vi "Save_Stats_for_Each_Block.vi"() -> (5 "Plug in titles":string[](array[string]), 7 "Plug in values":string[](array[string]))   [LabVIEW 2010]
uses:
  Globals/Meas_global.vi
  Globals/Plug_in_data_global.vi
  Globals/LDA_meas_global_1.vi
  <vilib>/Analysis/NI_AALBase.lvlib
panel:
  in  "Output Directory":path
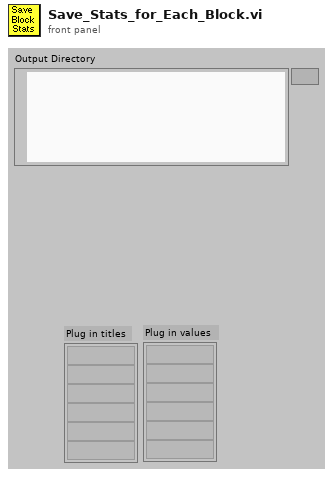
[diagram p1: front panel]
types:
  T1 = typedef "Analysis_info_cluster.ctl" = cluster{"Colour":u32, "Inst type":T2, "Inst name":string, "Symbol":string, "Code name":string, "Extra Info":string, "Inst Array":T3, "Index":i32, "Voltage Index":i32, "Extra Titles":string[], "Extra Values":string[]}
  T2 = typedef "Inst_type.ctl" = enum16{"Propeller anemometer", "Raw voltage", "Pressure Transducer", "Pitot-static tube", "Preston tube", "Hot wire", "Cross wire 1", "Cross wire 2", "Generic Linear", "Generic Polynomial", "Generic BackPoly", "Fast FID", "Thermocouple", "Cold wire", "Pulsed Wire", "LDA Vel", "LDA Tran time", "LDA Arr time"}
  T3 = typedef "Instrument_Array.ctl" = enum16{"PWA", "LDA", "Analogue"}
  T4 = enum32{"existing file", "new file", "new or existing file", "existing dir", "new dir", "new or existing dir", "existing file (use LLBs)", "new file (use LLBs)", "new or existing file (use LLBs)", "new or existing file or directory (use LLBs)"}
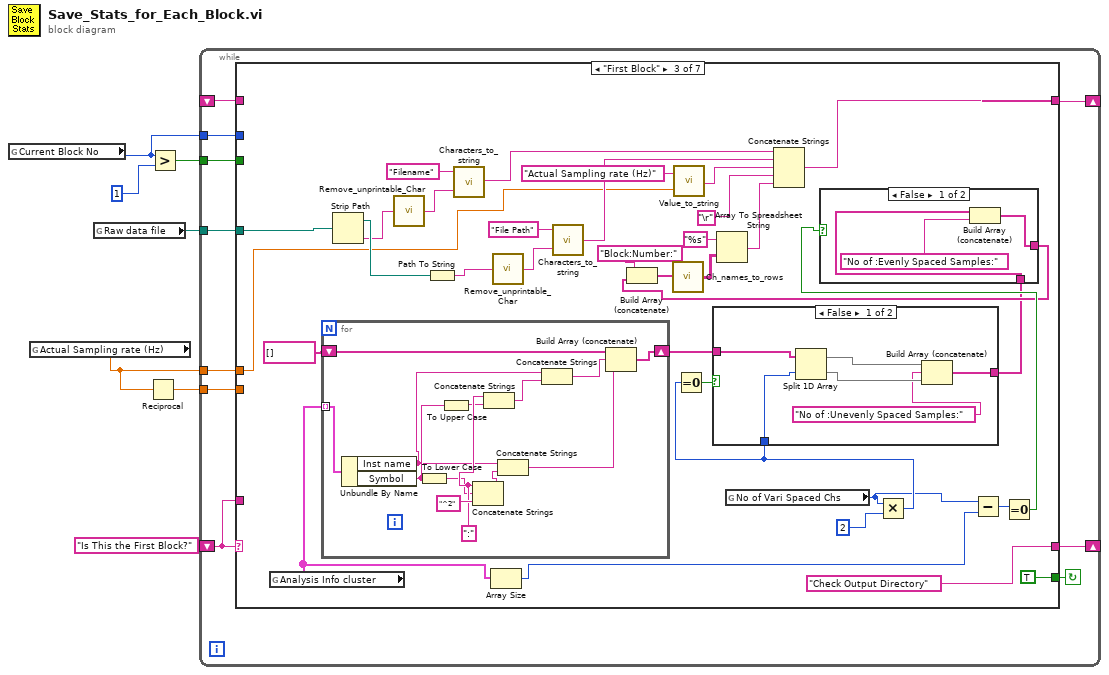
[diagram p0: block diagram]
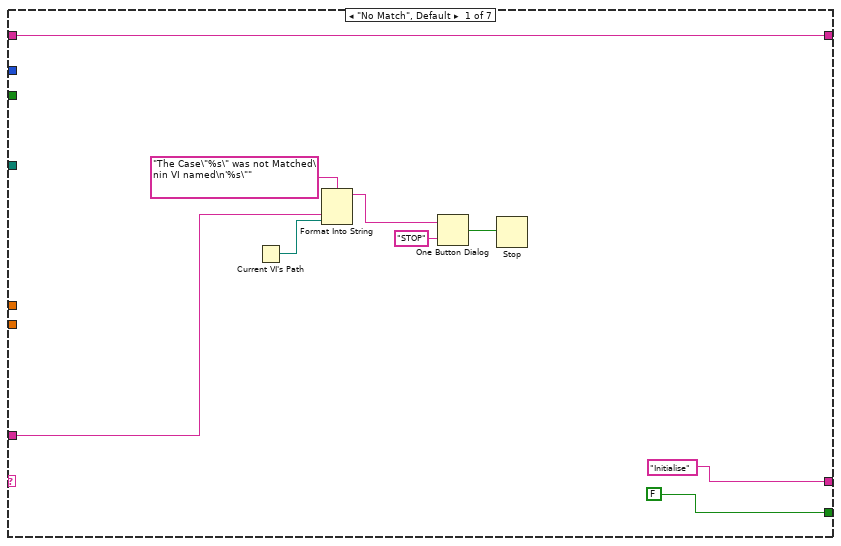
[diagram p2: hidden frame]
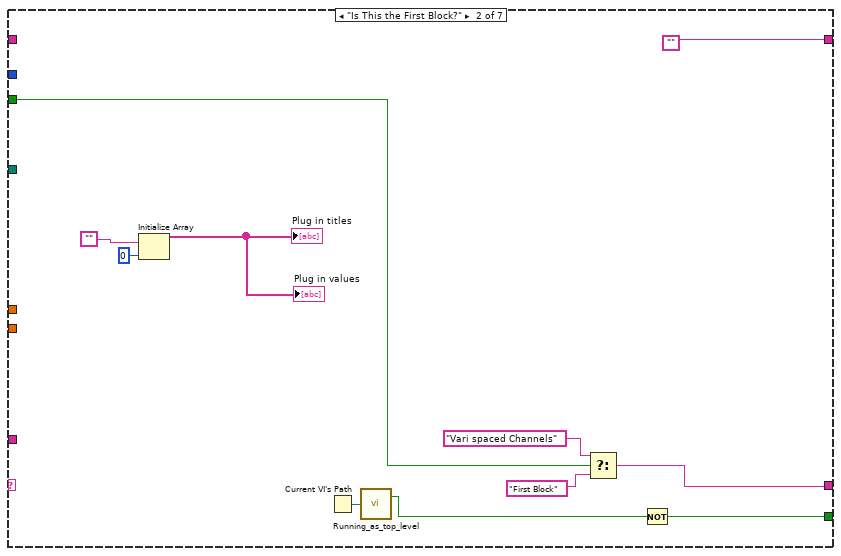
[diagram p3: hidden frame]
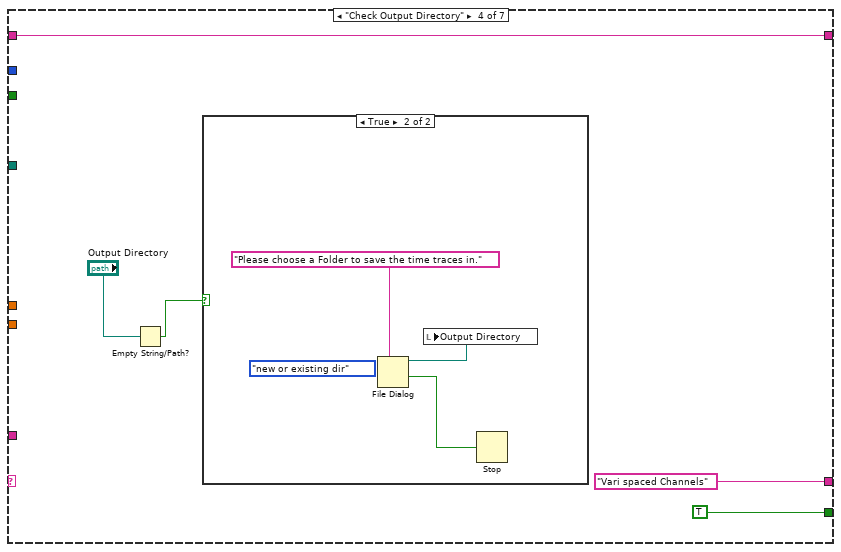
[diagram p6: hidden frame]
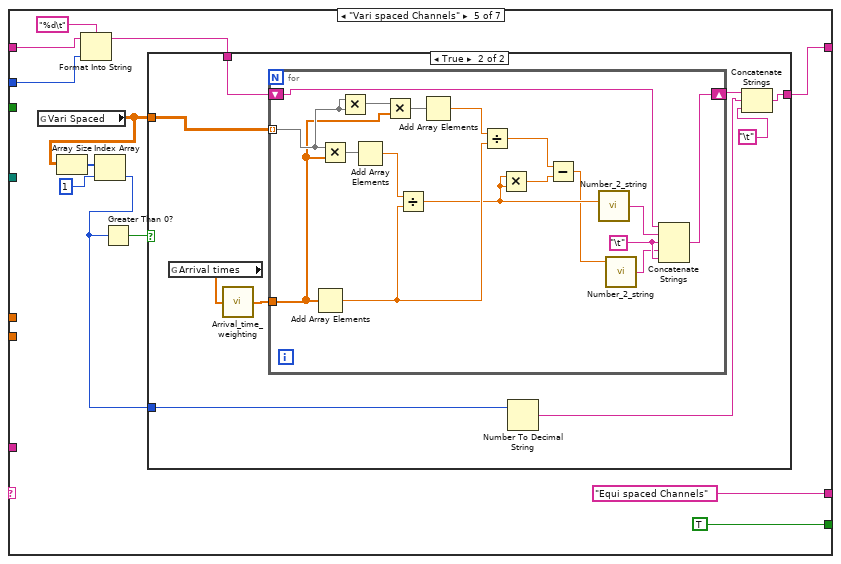
[diagram p8: hidden frame]
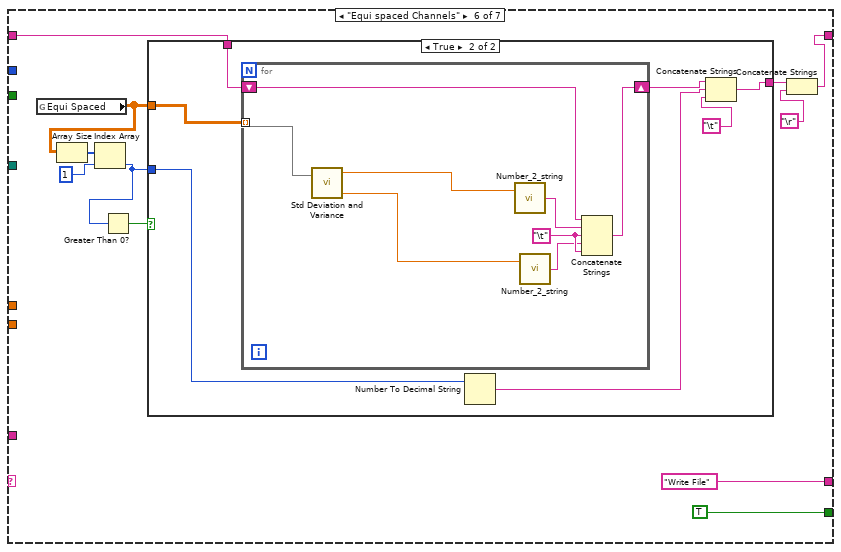
[diagram p10: hidden frame]
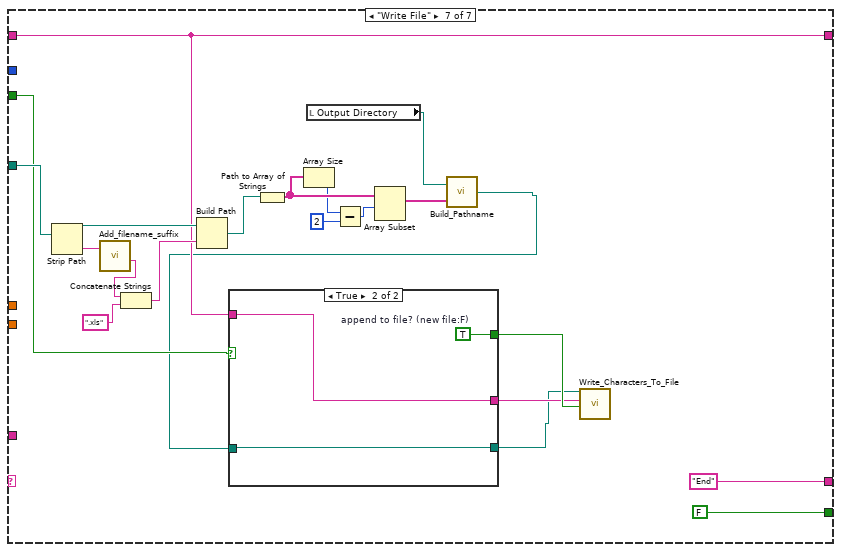
[diagram p12: hidden frame]
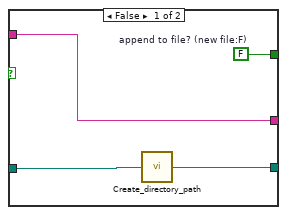
[diagram p13: hidden frame]
diagram:
  n1 = global read "Meas_global.vi" "Current Block No"() -> (w1:i32)
  n2 = global read "Meas_global.vi" "Actual Sampling rate (Hz)"() -> (w2:dbl)
  n3 = global read "Meas_global.vi" "Raw data file"() -> (w6:path)
  n4 = Reciprocal(x=w2) -> (1/x=w5:dbl)
  n5 = Greater?(x=w1, y=1) -> (0:w3:bool)
  n6 = while {
    shift-left: "Is This the First Block?" -> [w15]
    shift-right: [w16] -> _
    shift-right: [w13] -> _
    shift-left: _ -> [w12]
    tunnel: w6 -> [w14]
    tunnel: w5 -> [w11]
    tunnel: w3 -> [w10]
    tunnel: w2 -> [w9]
    tunnel: w1 -> [w8]
    stop <- w17 continue-if-true
    n7 = case shown="\"First Block\"" w15 {
      tunnel: [FALSE w27 TRUE TRUE TRUE TRUE FALSE] -> w17
      tunnel: ["Initialise" w36 "Check Output Directory" ("t") "Vari spaced Channels" ("t") "Equi spaced Channels" "Write File" "End" ("t")] -> w16
      tunnel: w15 -> [w21 _ _ _ _ _ _]
      tunnel: w14 -> [_ _ w60 _ _ _ w186]
      tunnel: [w18 "" w59 w98 w113 w145 w181] -> w13
      tunnel: w12 -> [w18 _ _ w98 w108 w151 w181]
      tunnel: w11 -> [_ _ _ _ _ _ _]
      tunnel: w10 -> [_ w34 _ _ _ _ w182]
      tunnel: w9 -> [_ _ w53 _ _ _ _]
      tunnel: w8 -> [_ _ _ _ w107 _ _]
      frame "No Match", Default {
        n8 = Current VI's Path() -> (path=w20:path)
        n9 = Format Into String(format string="The Case\"%s\" was not Matched\nin VI named\n'%s\"" ("Format String"), w21, w20) -> (resulting string=w24:string)  [unwired: 2 in, 1 out]
        n10 = One Button Dialog(message=w24, button name ("OK")="STOP") -> (true=w22:bool)
        n11 = Stop(stop? (T)=w22) -> ()
      }
      frame "Is This the First Block?" {
        n12 = Initialize Array("", 0) -> (→"Plug in values" →"Plug in titles":string[])
        n13 = Current VI's Path() -> (path=w29:path)
        n14 = call "Running_as_top_level.vi"("Vi path name"=w29) -> ("Top Level"=w28:bool)  [unwired: 1 out]
        n15 = Select(t="Vari spaced Channels", s=w34, f="First Block") -> (s? t:f=w36:string)
        n16 = Not(x=w28) -> (.not. x?=w27:bool)
      }
      frame "First Block" {
        n17 = global read "Meas_global.vi" "Analysis Info cluster"() -> (w45:T1[])
        n18 = for {
          tunnel: w45 -> [w95] mode=indexing
          shift-right: [w83] -> w50
          shift-left: string[] [] -> [w86]
          w91 = ":" ("string")
          n19 = Unbundle By Name(w95) -> ("Inst name"=w87:string, "Symbol"=w89:string)
          n20 = To Lower Case(string=w89) -> (all lower case string=w90:string)
          n21 = To Upper Case(1:w89) -> (0:w88:string)
          n22 = Concatenate Strings(w91, w90, "^2") -> (w93:string)
          n23 = Concatenate Strings(w91, w88) -> (w92:string)
          n24 = Concatenate Strings(w87, w93) -> (w84:string)
          n25 = Concatenate Strings(w87, w92) -> (w85:string)
          n26 = Build Array (concatenate)(w86, w85, w84) -> (w83:string[])
        }
        n27 = Strip Path(path=w60) -> (stripped path=w67:path, name=w63:string)
        n28 = call "Remove_unprintable_Char.vi"("Input String"=w63) -> ("Output String"=w64:string)
        n29 = Path To String(path=w67) -> (string=w68:string)
        n30 = call "Characters_to_string.vi"("Characters to write"=w64, "Label for characters"="Filename") -> ("Output string"=w69:string)
        n31 = Array Size(array=w45) -> (size(s)=w44:i32)
        n32 = call "Remove_unprintable_Char.vi"("Input String"=w68) -> ("Output String"=w65:string)
        n33 = call "Characters_to_string.vi"("Characters to write"=w65, "Label for characters"="File Path") -> ("Output string"=w70:string)
        n34 = call "Value_to_string.vi"("Value"=w53, "Label for value"="Actual Sampling rate (Hz)") -> ("Output string"=w57:string)  [unwired: 1 in]
        n35 = global read "Meas_global.vi" "No of Vari Spaced Chs"() -> (w46:i32)
        n36 = Multiply(x=w46, y=2) -> (x*y=w47:i32)
        n37 = Equal To 0?(x=w47) -> (x = 0?=w48:bool)
        n38 = case shown="False" w48 {
          tunnel: [w81 w82] -> w38
          tunnel: w50 -> [w80 w82]
          tunnel: w47 -> [w79 _]
          frame False {
            n39 = Split 1D Array(array=w80, index=w79) -> (first subarray=w78:string[], second subarray=w77:string[])
            n40 = Build Array (concatenate)(w78, "No of :Unevenly Spaced Samples:", w77) -> (w81:string[])
          }
          frame True {
          }
        }
        n41 = Subtract(x=w46, y=w44) -> (x-y=w41:i32)
        n42 = Equal To 0?(x=w41) -> (x = 0?=w40:bool)
        n43 = case shown="False" w40 {
          tunnel: [w72 w75] -> w39
          tunnel: w38 -> [w73 w75]
          frame False {
            n44 = Build Array (concatenate)(w73, "No of :Evenly Spaced Samples:") -> (w72:string[])
          }
          frame True {
          }
        }
        n45 = Build Array (concatenate)("Block:Number:", w39) -> (w43:string[])
        n46 = call "Ch_names_to_rows.vi"("Channel Names"=w43) -> ("3 Row names"=w42:string[][])
        n47 = Array To Spreadsheet String(array=w42, 3:"%s" ("format string")) -> (spreadsheet string=w55:string)  [unwired: 1 out]
        n48 = Concatenate Strings(w69, w70, w57, "\r", w55) -> (w59:string)
      }
      frame "Check Output Directory" {
        n49 = Empty String/Path?(string/path="Output Directory") -> (empty?=w99:bool)
        n50 = case shown="True" w99 {
          frame False {
          }
          frame True {
            (unwired) T4."new or existing dir" ("select mode (2)")
            n51 = File Dialog(7:"Please choose a Folder to save the time traces in." ("prompt")) -> (1:w102:bool, 3:w103:path)  [unwired: 1 in, 7 out]
            n52 = local write "Output Directory"(w103) -> ()
            n53 = Stop(stop? (T)=w102) -> ()
          }
        }
      }
      frame "Vari spaced Channels" {
        n54 = global read "Plug_in_data_global.vi" "Vari Spaced"() -> (w112:dbl[][])
        n55 = Array Size(array=w112) -> (size(s)=w110:i32[])
        n56 = Format Into String(format string="%d\t", initial string=w108, w107) -> (resulting string=w105:string)  [unwired: 1 in, 1 out]
        n57 = Index Array(array=w110, index=1) -> (element=w104:i32)
        n58 = Greater Than 0?(x=w104) -> (x > 0?=w109:bool)
        n59 = case shown="True" w109 {
          tunnel: w112 -> [_ w124]
          tunnel: w105 -> [w116 w122]
          tunnel: [w116 w119] -> w113
          tunnel: w104 -> [_ w121]
          frame False {
          }
          frame True {
            n60 = global read "LDA_meas_global_1.vi" "Arrival times"() -> (w125:dbl[])
            n61 = call "Arrival_time_weighting.vi"("Arrival times"=w125) -> ("Weighting"=w123:dbl[])
            n62 = for {
              tunnel: w124 -> [w140] mode=indexing
              tunnel: w123 -> [w138]
              shift-right: [w131] -> w120
              shift-left: w122 -> [w132]
              w130 = "\t"
              n63 = Add Array Elements(numeric array=w138) -> (sum=w135:dbl)
              n64 = Multiply(x=w140, y=w138) -> (x*y=w142:dbl[])
              n65 = Multiply(x=w140, y=w140) -> (x*y=w139:dbl[])
              n66 = Add Array Elements(numeric array=w142) -> (sum=w141:dbl)
              n67 = Multiply(x=w139, y=w138) -> (x*y=w137:dbl[])
              n68 = Divide(x=w141, y=w135) -> (x/y=w129:dbl)
              n69 = Add Array Elements(numeric array=w137) -> (sum=w136:dbl)
              n70 = Divide(x=w136, y=w135) -> (x/y=w134:dbl)
              n71 = Multiply(x=w129, y=w129) -> (x*y=w133:dbl)
              n72 = Subtract(x=w134, y=w133) -> (x-y=w128:dbl)
              n73 = call "Number_2_string.vi"("number"=w129) -> ("String"=w126:string)  [unwired: 1 in]
              n74 = call "Number_2_string.vi"("number"=w128) -> ("String"=w127:string)  [unwired: 1 in]
              n75 = Concatenate Strings(w132, w126, w130, w127, w130) -> (w131:string)
            }
            n76 = Number To Decimal String(number=w121) -> (decimal integer string=w118:string)  [unwired: 1 out]
            n77 = Concatenate Strings(w120, w118, "\t") -> (w119:string)
          }
        }
      }
      frame "Equi spaced Channels" {
        n78 = global read "Plug_in_data_global.vi" "Equi Spaced"() -> (w150:dbl[][])
        n79 = Array Size(array=w150) -> (size(s)=w148:i32[])
        n80 = Index Array(array=w148, index=1) -> (element=w143:i32)
        n81 = Greater Than 0?(x=w143) -> (x > 0?=w147:bool)
        n82 = case shown="True" w147 {
          tunnel: w150 -> [_ w161]
          tunnel: w151 -> [w154 w160]
          tunnel: [w154 w157] -> w146
          tunnel: w143 -> [_ w156]
          frame False {
          }
          frame True {
            n83 = for {
              tunnel: w161 -> [w166] mode=indexing
              shift-right: [w169] -> w158
              shift-left: w160 -> [w167]
              w168 = "\t"
              n84 = call <vilib>:"Std Deviation and Variance.vi"("X"=w166) -> ("mean"=w165:dbl, "variance"=w164:dbl)  [unwired: 1 in, 1 out]
              n85 = call "Number_2_string.vi"("number"=w165) -> ("String"=w162:string)  [unwired: 1 in]
              n86 = call "Number_2_string.vi"("number"=w164) -> ("String"=w163:string)  [unwired: 1 in]
              n87 = Concatenate Strings(w167, w162, w168, w163, w168) -> (w169:string)
            }
            n88 = Number To Decimal String(number=w156) -> (decimal integer string=w155:string)  [unwired: 1 out]
            n89 = Concatenate Strings(w158, w155, "\t") -> (w157:string)
          }
        }
        n90 = Concatenate Strings(w146, "\r") -> (w145:string)
      }
      frame "Write File" {
        n91 = Strip Path(path=w186) -> (stripped path=w188:path, name=w171:string)
        n92 = call "Add_filename_suffix.vi"("Filename"=w171) -> ("Base name"=w170:string)  [unwired: 1 in, 3 out]
        n93 = Concatenate Strings(w170, ".xls" ("Substring")) -> (w189:string)
        n94 = Build Path(base path=w188, name or relative path=w189) -> (appended path=w187:path)
        n95 = Path to Array of Strings(0:w187) -> (2:w178:string[])  [unwired: 1 out]
        n96 = Array Size(array=w178) -> (size(s)=w177:i32)
        n97 = local read "Output Directory"() -> (w173:path)
        n98 = Subtract(x=w177, y=2) -> (x-y=w175:i32)
        n99 = Array Subset(array=w178, index=w175) -> (w174:string[])  [unwired: 1 in]
        n100 = call "Build_Pathname.vi"("Output Array"=w174, "Pathname"=w173) -> ("Appended path"=w172:path)
        n101 = case shown="True" w182 {
          tunnel: [w191 w197] -> w184
          tunnel: w181 -> [w191 w197]
          tunnel: [w194 w196] -> w185
          tunnel: w172 -> [w193 w195]
          tunnel: [w192 w195] -> w183
          frame False {
            w194 = FALSE  # append to file? (new file:F)
            n102 = call "Create_directory_path.vi"("Path name"=w193) -> ("Path name Out"=w192:path)
          }
          frame True {
            w196 = TRUE  # append to file? (new file:F)
          }
        }
        n103 = call "Write_Characters_To_File.vi"("file path (dialog if empty)"=w183, "character string"=w184, "append to file? (new file:F)"=w185) -> ()  [unwired: 2 in, 4 out]
      }
    }
  }
